vi "LabVIEW GEMM And Operations.vi"(11 "dimension size":i32=20000) -> (3 "LabVIEW Time":dbl)   [LabVIEW 2020]
uses:
  <vilib>/Analysis/BLAS.llb/dgemm - General Matrix-Matrix Product (DBL).vi
  <vilib>/Analysis/Matrix/Numeric/Conversions/Matrix To Array - RM.vi
  <vilib>/Analysis/NI_AALBLAS.lvlib
  <vilib>/Analysis/Matrix/NI_Matrix.lvlib
  <vilib>/Analysis/NI_AALBase.lvlib
panel:
  out "max value 2":dbl
  out "max value":dbl
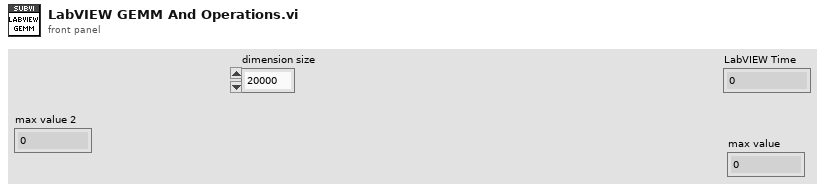
[diagram p1: front panel]
types:
  T1 = typedef "NI_Matrix.lvlib/RealMatrix.ctl" = dbl[][]
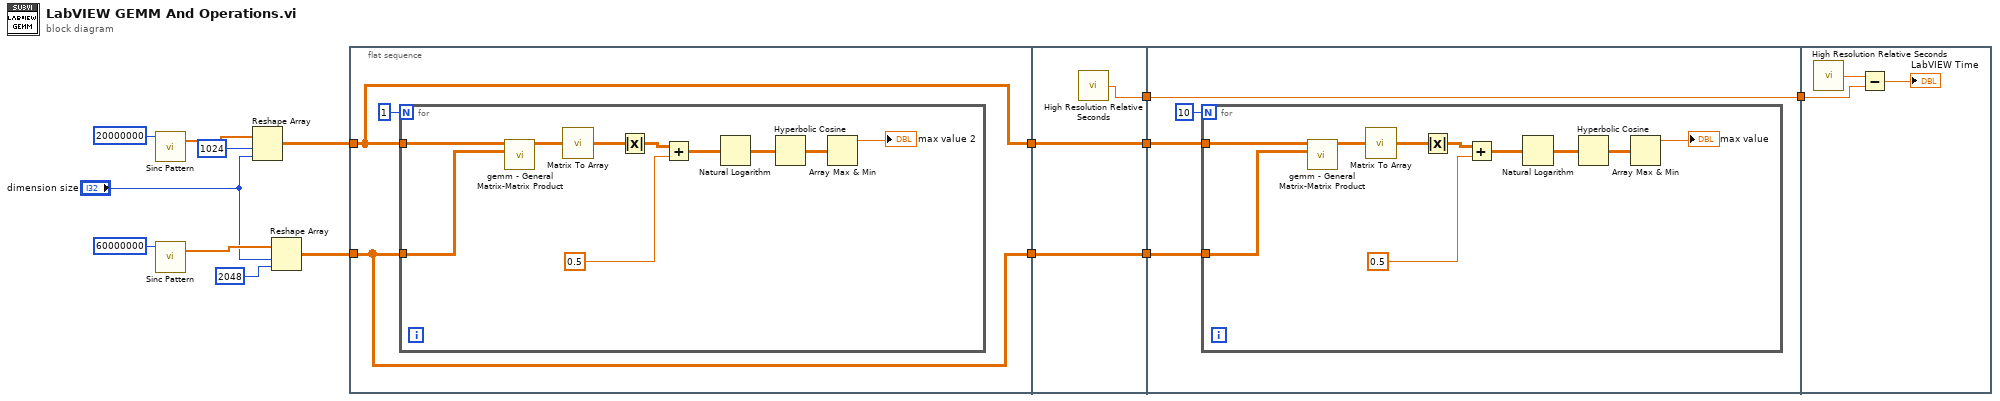
[diagram p0: block diagram]
diagram:
  n1 = call <vilib>:"Sinc Pattern.vi"("samples"=20000000) -> ("Sinc Pattern"=w7:dbl[])  [unwired: 3 in, 1 out]
  n2 = call <vilib>:"Sinc Pattern.vi"("samples"=60000000) -> ("Sinc Pattern"=w6:dbl[])  [unwired: 3 in, 1 out]
  n3 = Reshape Array(w7, 1024 ("dimension size"), "dimension size") -> (w8:dbl[][])
  n4 = Reshape Array(w6, "dimension size", 2048 ("dimension size")) -> (w4:dbl[][])
  n5 = flat-sequence {
    tunnel: w4 -> [w16]
    tunnel: w8 -> [w17]
    tunnel: [w17] -> w2
    tunnel: [w16] -> w1
    tunnel: [w31] -> w13
    tunnel: [w30] -> w9
    tunnel: [w29] -> w5
    tunnel: w2 -> [w30]
    tunnel: w1 -> [w29]
    tunnel: w13 -> [w35]
    tunnel: [w35] -> w12
    tunnel: w9 -> [w34]
    tunnel: w5 -> [w33]
    tunnel: w12 -> [w47]
    frame #0 {
      n6 = for {
        N: 1 -> [_]
        tunnel: w17 -> [w20]
        tunnel: w16 -> [w19]
        n7 = call-poly <vilib>:"gemm - General Matrix-Matrix Product.vi"("B"=w19, "A"=w20) -> ("dgemm"=w28:T1)  [unwired: 8 in, 1 out]
        n8 = call-poly <vilib>:"Matrix To Array.vi"("Real Matrix"=w28) -> ("Real 2D Array"=w22:dbl[][])
        n9 = Absolute Value ("Absolute Value.vi")(x=w22) -> (abs(x)=w25:dbl[][])
        n10 = Add ("Add.vi")(x=w25, y=0.5) -> (x+y=w26:dbl[][])
        n11 = Natural Logarithm ("Natural Logarithm.vi")(1:w26) -> (0:w24:dbl[][])
        n12 = Hyperbolic Cosine(1:w24) -> (0:w23:dbl[][])
        n13 = Array Max & Min(array=w23) -> (max value=→"max value 2":dbl)  [unwired: 3 out]
      }
    }
    frame #1 {
      n14 = call <vilib>:"High Resolution Relative Seconds.vi"() -> ("relative seconds"=w31:dbl)
    }
    frame #2 {
      n15 = for {
        N: 10 -> [_]
        tunnel: w34 -> [w37]
        tunnel: w33 -> [w36]
        n16 = call-poly <vilib>:"gemm - General Matrix-Matrix Product.vi"("B"=w36, "A"=w37) -> ("dgemm"=w45:T1)  [unwired: 8 in, 1 out]
        n17 = call-poly <vilib>:"Matrix To Array.vi"("Real Matrix"=w45) -> ("Real 2D Array"=w39:dbl[][])
        n18 = Absolute Value ("Absolute Value.vi")(x=w39) -> (abs(x)=w42:dbl[][])
        n19 = Add ("Add.vi")(x=w42, y=0.5) -> (x+y=w43:dbl[][])
        n20 = Natural Logarithm ("Natural Logarithm.vi")(1:w43) -> (0:w41:dbl[][])
        n21 = Hyperbolic Cosine(1:w41) -> (0:w40:dbl[][])
        n22 = Array Max & Min(array=w40) -> (max value=→"max value":dbl)  [unwired: 3 out]
      }
    }
    frame #3 {
      n23 = call <vilib>:"High Resolution Relative Seconds.vi"() -> ("relative seconds"=w48:dbl)
      n24 = Subtract(x=w48, y=w47) -> (x-y=→"LabVIEW Time":dbl)
    }
  }
